vi "Read CSM States.vi"(8 "error in (no error)":errorcluster, 11 "CSM-Helper in":refnum<class "CSM-Helper.lvclass">) -> (0 "error out":errorcluster, 2 "Value":string[](array[string]), 3 "CSM-Helper out":refnum<class "CSM-Helper.lvclass">)   [LabVIEW 2020, in "CSM-Helper.lvclass"]
uses:
  CSM-Helper.lvclass
  CSM-Helper.lvclass/CSM-Helper.ctl
  <userlib>/_OpenG.lib/string/string.llb/Trim Whitespace (String Array)__ogtk.vi
  <userlib>/_OpenG.lib/array/array.llb/Filter 1D Array (String)__ogtk.vi
  <userlib>/_OpenG.lib/array/array.llb/Filter 1D Array with Scalar (String)__ogtk.vi
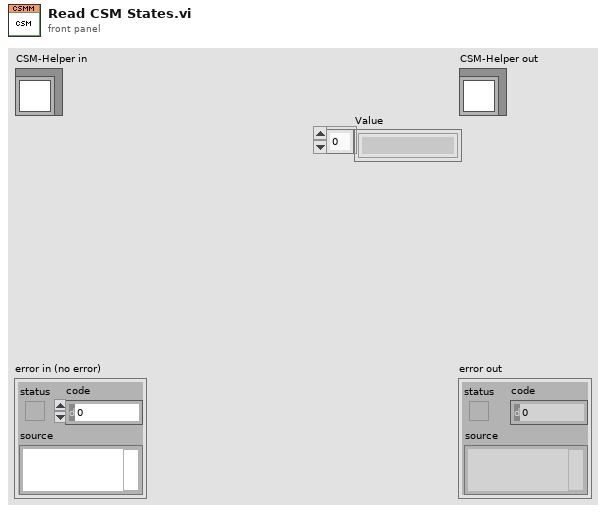
[diagram p1: front panel]
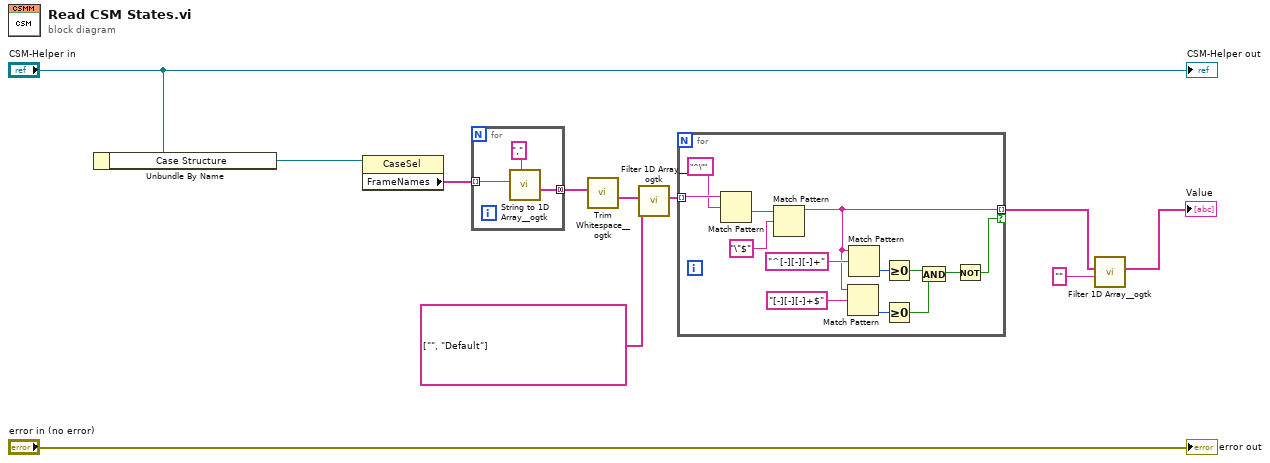
[diagram p0: block diagram]
diagram:
  n1 = Unbundle By Name("CSM-Helper in") -> ("Case Structure"=w5:refnum<vi>)
  n2 = property on="Property Node" class="CaseSel"(reference=w5) -> ("FrameNames"=w11:string[])  [unwired: 1 in, 2 out]
  n3 = for {
    tunnel: w11 -> [w14] mode=indexing
    tunnel: [w12] -> w10 mode=concatenating
    n4 = call <userlib>:"String to 1D Array__ogtk.vi"("delimiter (Tab)"=",", "string"=w14) -> ("Array of Strings"=w12:string[])  [unwired: 9 in]
  }
  n5 = call-poly <userlib>:"Trim Whitespace__ogtk.vi"("String in"=w10) -> ("String out"=w9:string[])  [unwired: 6 in]
  n6 = call-poly <userlib>:"Filter 1D Array__ogtk.vi"("items to filter"=string[] ["", "Default"], "array"=w9) -> ("filtered array"=w7:string[])  [unwired: 4 in, 1 out]
  n7 = for {
    tunnel: w7 -> [w27] mode=indexing
    tunnel: [w15] -> w3 mode=indexing if=w16
    n8 = Match Pattern(string=w27, regular expression="^\"") -> (after substring=w25:string)  [unwired: 1 in, 3 out]
    n9 = Match Pattern(string=w25, regular expression="\"$") -> (before substring=w15:string)  [unwired: 1 in, 3 out]
    n10 = Match Pattern(string=w15, regular expression="[-][-][-]+$") -> (offset past match=w20:i32)  [unwired: 1 in, 3 out]
    n11 = Match Pattern(string=w15, regular expression="^[-][-][-]+") -> (offset past match=w21:i32)  [unwired: 1 in, 3 out]
    n12 = Greater Or Equal To 0?(x=w21) -> (x >= 0?=w19:bool)
    n13 = Greater Or Equal To 0?(x=w20) -> (x >= 0?=w18:bool)
    n14 = And(x=w19, y=w18) -> (x .and. y?=w17:bool)
    n15 = Not(x=w17) -> (.not. x?=w16:bool)
  }
  n16 = call-poly <userlib>:"Filter 1D Array__ogtk.vi"("items to filter"="" ("String"), "array"=w3) -> ("filtered array"=→"Value":string[])  [unwired: 4 in, 1 out]
  "error out" <- "error in (no error)"
  "CSM-Helper out" <- "CSM-Helper in"
